vi "Create_Block_From_type.vi"(10 "Numeric":dbl) -> (3 "Cluster":T1 {"orientaion" items=["up", "down", "left", "right"]; "type" items=["t", "rl", "ll", "rz", "lz", "square", "line"]})   [LabVIEW 2015]
uses:
  block.ctl
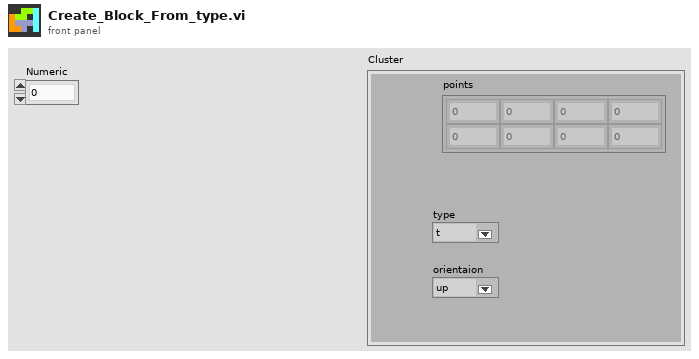
[diagram p1: front panel]
types:
  T1 = typedef "block.ctl" = cluster{"points":dbl[][], "type":u16, "orientaion":u16}
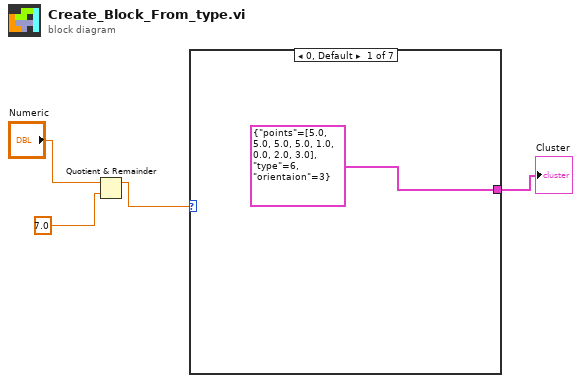
[diagram p0: block diagram]
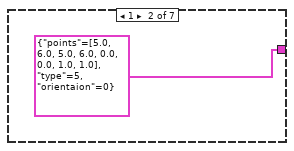
[diagram p2: hidden frame]
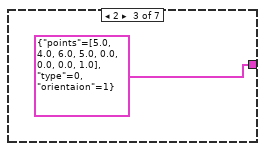
[diagram p3: hidden frame]
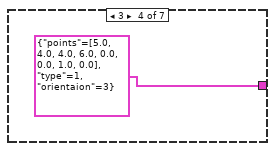
[diagram p4: hidden frame]
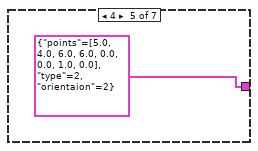
[diagram p5: hidden frame]
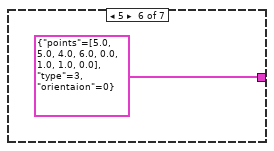
[diagram p6: hidden frame]
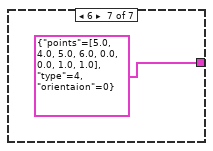
[diagram p7: hidden frame]
diagram:
  n1 = Quotient & Remainder(x="Numeric", y=7.0) -> (x-y*floor(x/y)=w3:dbl)  [unwired: 1 out]
  n2 = case shown="0, Default" w3 {
    tunnel: [T1 {"points"=[[5.0, 5.0, 5.0, 5.0], [1.0, 0.0, 2.0, 3.0]], "type"=6, "orientaion"=3} ("Cluster") T1 {"points"=[[5.0, 6.0, 5.0, 6.0], [0.0, 0.0, 1.0, 1.0]], "type"=5, "orientaion"=0} ("Cluster") T1 {"points"=[[5.0, 4.0, 6.0, 5.0], [0.0, 0.0, 0.0, 1.0]], "type"=0, "orientaion"=1} ("Cluster") T1 {"points"=[[5.0, 4.0, 4.0, 6.0], [0.0, 0.0, 1.0, 0.0]], "type"=1, "orientaion"=3} ("Cluster") T1 {"points"=[[5.0, 4.0, 6.0, 6.0], [0.0, 0.0, 1.0, 0.0]], "type"=2, "orientaion"=2} ("Cluster") T1 {"points"=[[5.0, 5.0, 4.0, 6.0], [0.0, 1.0, 1.0, 0.0]], "type"=3, "orientaion"=0} ("Cluster") T1 {"points"=[[5.0, 4.0, 5.0, 6.0], [0.0, 0.0, 1.0, 1.0]], "type"=4, "orientaion"=0} ("Cluster")] -> w4
    frame 0, Default {
    }
    frame 1 {
    }
    frame 2 {
    }
    frame 3 {
    }
    frame 4 {
    }
    frame 5 {
    }
    frame 6 {
    }
  }
  "Cluster" <- w4
